vi "Configure Measurement_.vi"(8 "error in (no error)":errorcluster, 10 "Function (0: Cp-D)":T1, 11 "Agilent E4980 in":refnum<class "Agilent E4980.lvclass">) -> (0 "error out":errorcluster, 3 "Agilent E4980 out":refnum<class "Agilent E4980.lvclass">)   [LabVIEW 2020, in "Agilent E4980.lvclass"]
uses:
  Agilent E4980.lvclass
  C:/Sandbox/RF Bench/Source Code/WiSpry Test Framework/Instruments/Instrument.lvclass
  Controls/Function.ctl
  Instrument.lvclass/Instrument.ctl
  Instrument.lvclass
  <instrlib>/Agilent E4980/Agilent E4980.lvlib
  LCR Meter.lvclass
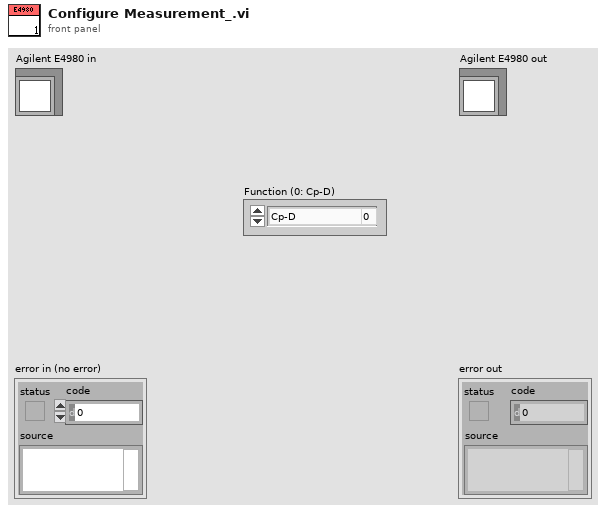
[diagram p1: front panel]
types:
  T1 = typedef "LCR Meter.lvclass/Function.ctl" = enum16{"Cp-D", "Cp-Q", "Cp-G", "Cp-Rp", "Cs-D", "Cs-Q", "Cs-Rs", "Lp-D", "Lp-Q", "Lp-G", "Lp-Rp", "Lp-Rdc", "Ls-D", "Ls-Q", "Ls-Rs", "Ls-Rdc", "R-X", "Z-thd", "Z-thr", "G-B", "Y-thd", "Y-thr", "Vdc-Idc"}
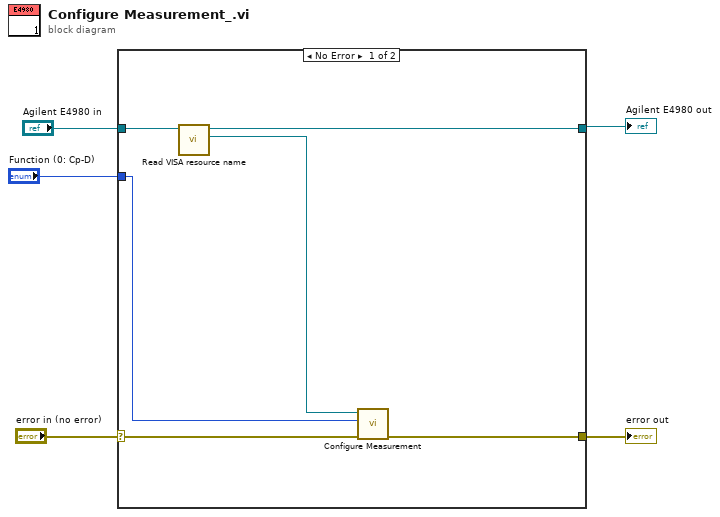
[diagram p0: block diagram]
diagram:
  n1 = case shown="No Error" "error in (no error)" {
    selector: "error in (no error)" -> [w9 w13]
    tunnel: [w7 w13] -> w4
    tunnel: [w10 w12] -> w3
    tunnel: "Agilent E4980 in" -> [w11 w12]
    tunnel: "Function (0: Cp-D)" -> [w6 _]
    frame No Error {
      n2 = call "Read VISA resource name.vi"("Instrument in"=w11) -> ("VISA resource name"=w8:refnum<visa-resource-name>, "Instrument out"=w10:refnum<class "Agilent E4980.lvclass">)  [unwired: 9 in]
      n3 = call <instrlib>:"Configure Measurement.vi"("error in (no error)"=w9, "Function (0: Cp-D)"=w6, "VISA resource name"=w8) -> ("error out"=w7:errorcluster)  [unwired: 7 in, 1 out]
    }
    frame Error {
    }
  }
  "error out" <- w4
  "Agilent E4980 out" <- w3
